vi "ClusterWayToSendClientSide.vi"() -> ()   [LabVIEW 2019]
panel:
  out "Full Name":string
  out "Single or not":bool
  out "Age from server side":dbl
  in  "type":T1
  in  "Stop from Client side":bool
  out "error out":errorcluster
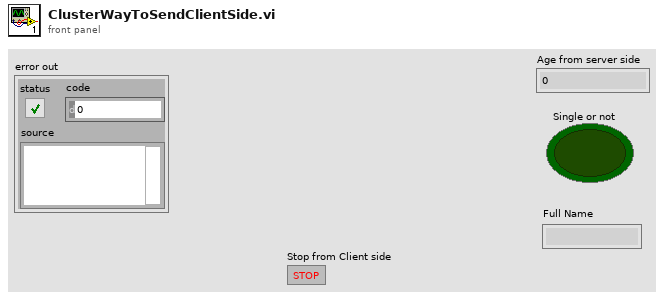
[diagram p1: front panel]
types:
  T1 = cluster{"Age ":dbl, "Is Single":bool, "Full Name ":string}
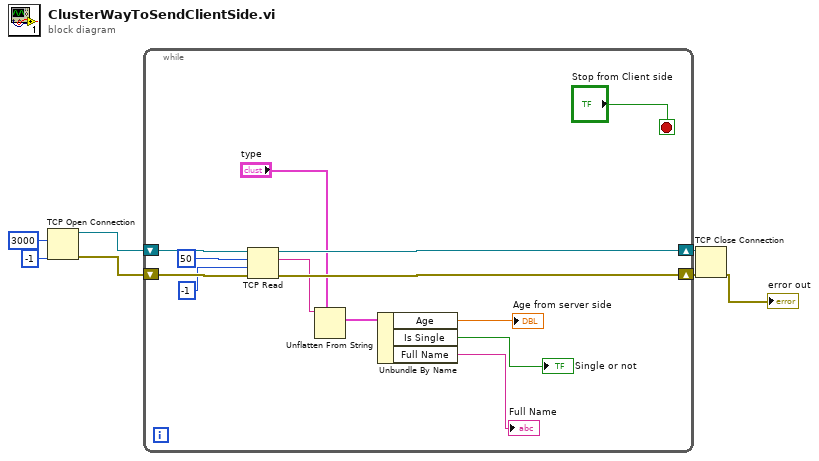
[diagram p0: block diagram]
diagram:
  n1 = TCP Open Connection(remote port or service name=u16 3000, timeout ms (60000)=-1) -> (connection ID=w5:refnum<k5>, error out=w4:errorcluster)  [unwired: 3 in]
  n2 = while {
    shift-right: [w17] -> w2
    shift-left: w5 -> [w20]
    shift-right: [w18] -> w3
    shift-left: w4 -> [w19]
    stop <- "Stop from Client side" stop-if-true
    n3 = TCP Read(connection ID=w20, bytes to read=50, error in (no error)=w19, 9:-1 ("timeout ms (25000)")) -> (connection ID out=w17:refnum<k5>, data out=w13:string, error out=w18:errorcluster)  [unwired: 1 in]
    n4 = Unflatten From String(type="type", binary string=w13) -> (value=w11:T1)  [unwired: 3 in, 2 out]
    n5 = Unbundle By Name(w11) -> ("Age"=→"Age from server side":dbl, "Is Single"=→"Single or not":bool, "Full Name"=→"Full Name":string)
  }
  n6 = TCP Close Connection(connection ID=w2, error in (no error)=w3) -> (error out=→"error out":errorcluster)  [unwired: 1 in, 1 out]
